vi "TestExec.Append Fault Code Prefix_V2.vi"(7 "Positive(F)\\Negative(T)":bool, 9 "FaultCode":i32, 10 "FaultCode Prefix":i32) -> (1 "New Fault Code":i32)   [LabVIEW 2019]
panel:
  out "StrOutput":string
  out "StrCode":string
  out "StrPrefix":string
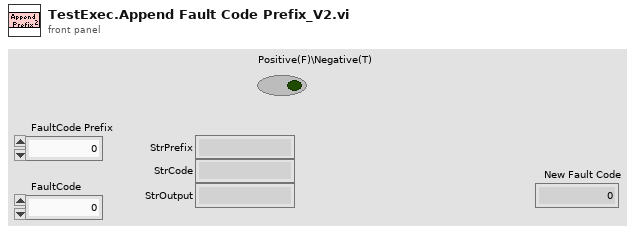
[diagram p1: front panel]
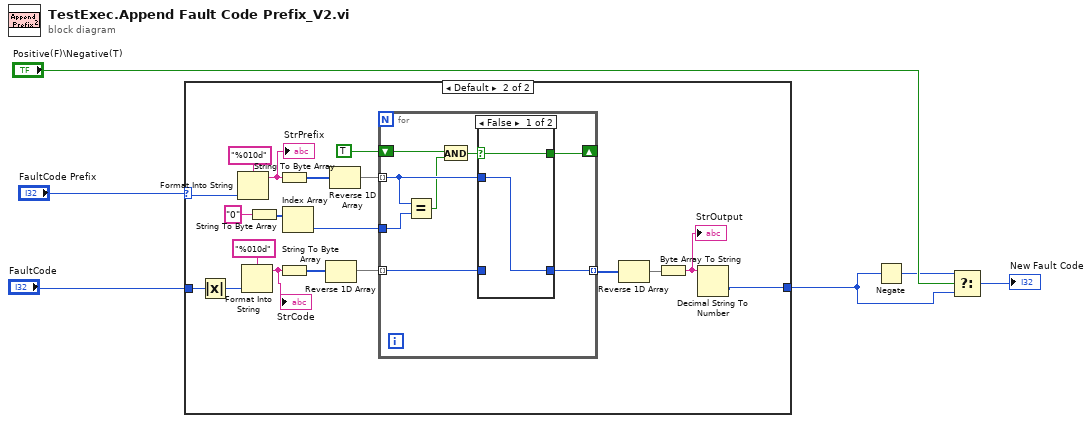
[diagram p0: block diagram]
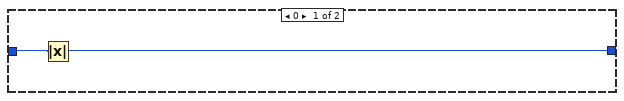
[diagram p2: hidden frame]
diagram:
  n1 = case shown="Default" "FaultCode Prefix" {
    selector: "FaultCode Prefix" -> [_ w23]
    tunnel: "FaultCode" -> [w8 w27]
    tunnel: [w7 w19] -> w2
    frame 0 {
      n2 = Absolute Value(x=w8) -> (abs(x)=w7:i32)
    }
    frame Default {
      n3 = Absolute Value(x=w27) -> (abs(x)=w24:i32)
      n4 = Format Into String(format string="%010d", w23) -> (resulting string=w18:string)  [unwired: 2 in, 1 out]
      "StrPrefix" <- w18
      n5 = Format Into String(format string="%010d", w24) -> (resulting string=w17:string)  [unwired: 2 in, 1 out]
      "StrCode" <- w17
      n6 = String To Byte Array(string="0") -> (unsigned byte array=w21:u8[])
      n7 = String To Byte Array(string=w18) -> (unsigned byte array=w14:u8[])
      n8 = String To Byte Array(string=w17) -> (unsigned byte array=w13:u8[])
      n9 = Index Array(array=w21) -> (element=w20:u8)  [unwired: 1 in]
      n10 = Reverse 1D Array(array=w13) -> (reversed array=w10:u8[])
      n11 = Reverse 1D Array(array=w14) -> (reversed array=w15:u8[])
      n12 = for {
        tunnel: w15 -> [w34] mode=indexing
        tunnel: w10 -> [w33] mode=indexing
        tunnel: w20 -> [w35]
        tunnel: [w32] -> w12 mode=indexing
        shift-right: [w28] -> _
        shift-left: TRUE -> [w31]
        n13 = Equal?(x=w34, y=w35) -> (x = y?=w30:bool)
        n14 = And(x=w31, y=w30) -> (x .and. y?=w29:bool)
        n15 = case shown="False" w29 {
          selector: w29 -> [w36 w38]
          tunnel: w34 -> [w37 _]
          tunnel: w33 -> [_ w39]
          tunnel: [w37 w39] -> w32
          tunnel: [w36 w38] -> w28
          frame False {
          }
          frame True {
          }
        }
      }
      n16 = Reverse 1D Array(array=w12) -> (reversed array=w11:u8[])
      n17 = Byte Array To String(unsigned byte array=w11) -> (string=w16:string)
      "StrOutput" <- w16
      n18 = Decimal String To Number(string=w16) -> (number=w19:i32)  [unwired: 2 in, 1 out]
    }
  }
  n19 = Negate(x=w2) -> (-x=w4:i32)
  n20 = Select(t=w4, s="Positive(F)\\Negative(T)", f=w2) -> (s? t:f=→"New Fault Code":i32)
